vi "Node - Runtime Type Cast.vi"(8 "error in (no error)":errorcluster, 11 "Node Data In":T1) -> (0 "error out":errorcluster, 2 "Buffer Offset Out":u64, 3 "Node Data Out":T1)   [LabVIEW 2016, in "PXImc Router.lvlib"]
uses:
  Controls/Node Data.ctl
  <vilib>/NI Veristand/VeriStand Data/Byte Buffer/Byte Buffer.lvclass
  Controls/Node/Node - PXImc Parameters.ctl
  Controls/Node/Transfer Data.ctl
  Controls/Node/Node Ch Properties.ctl
  Controls/Data Type.ctl
  <vilib>/NI Veristand/VeriStand Data/Byte Buffer/Byte Buffer.lvclass/Byte Buffer.ctl
  <vilib>/NI Veristand/VeriStand Data/Type Conversion/Type Conversion.From Double (Boolean).vi
  <vilib>/NI Veristand/VeriStand Data/Byte Buffer/Byte Buffer.Write (Boolean).vi
  <vilib>/NI Veristand/VeriStand Data/Type Conversion/Type Conversion.From Double (SGL).vi
  <vilib>/NI Veristand/VeriStand Data/Byte Buffer/Byte Buffer.Write (SGL).vi
  <vilib>/NI Veristand/VeriStand Data/Byte Buffer/Byte Buffer.Write (DBL).vi
  <vilib>/NI Veristand/VeriStand Data/Type Conversion/Type Conversion.From Double (I8).vi
  <vilib>/NI Veristand/VeriStand Data/Byte Buffer/Byte Buffer.Write (I8).vi
  <vilib>/NI Veristand/VeriStand Data/Type Conversion/Type Conversion.From Double (I16).vi
  <vilib>/NI Veristand/VeriStand Data/Byte Buffer/Byte Buffer.Write (I16).vi
  <vilib>/NI Veristand/VeriStand Data/Type Conversion/Type Conversion.From Double (I32).vi
  <vilib>/NI Veristand/VeriStand Data/Byte Buffer/Byte Buffer.Write (I32).vi
  <vilib>/NI Veristand/VeriStand Data/Type Conversion/Type Conversion.From Double (I64).vi
  <vilib>/NI Veristand/VeriStand Data/Byte Buffer/Byte Buffer.Write (I64).vi
  <vilib>/NI Veristand/VeriStand Data/Type Conversion/Type Conversion.From Double (U8).vi
  <vilib>/NI Veristand/VeriStand Data/Byte Buffer/Byte Buffer.Write (U8).vi
  <vilib>/NI Veristand/VeriStand Data/Type Conversion/Type Conversion.From Double (U16).vi
  <vilib>/NI Veristand/VeriStand Data/Byte Buffer/Byte Buffer.Write (U16).vi
  <vilib>/NI Veristand/VeriStand Data/Type Conversion/Type Conversion.From Double (U32).vi
  <vilib>/NI Veristand/VeriStand Data/Byte Buffer/Byte Buffer.Write (U32).vi
  <vilib>/NI Veristand/VeriStand Data/Type Conversion/Type Conversion.From Double (U64).vi
  <vilib>/NI Veristand/VeriStand Data/Byte Buffer/Byte Buffer.Write (U64).vi
  <vilib>/NI Veristand/VeriStand Data/Byte Buffer/Byte Buffer.Write (String).vi
  <vilib>/NI Veristand/VeriStand Data/Byte Buffer/Byte Buffer.Subset.Set.vi
  <vilib>/NI Veristand/VeriStand Data/Byte Buffer/Byte Buffer.Get Buffer Pointer.vi
  <vilib>/NI Veristand/VeriStand Data/Byte Buffer/Byte Buffer.Get Buffer Size.vi
  <vilib>/NI Veristand/VeriStand Data/Memory Management/Memory Management.MoveByteBlock.Read (String).vi
  <vilib>/NI Veristand/VeriStand Data/Byte Buffer/Byte Buffer.Get Byte Order.vi
  <vilib>/NI Veristand/VeriStand Data/Memory Management/Memory Management.Handle Return.vi
  PXImc Router.lvlib
  <vilib>/NI Veristand/VeriStand Data/VeriStand Data.lvlib
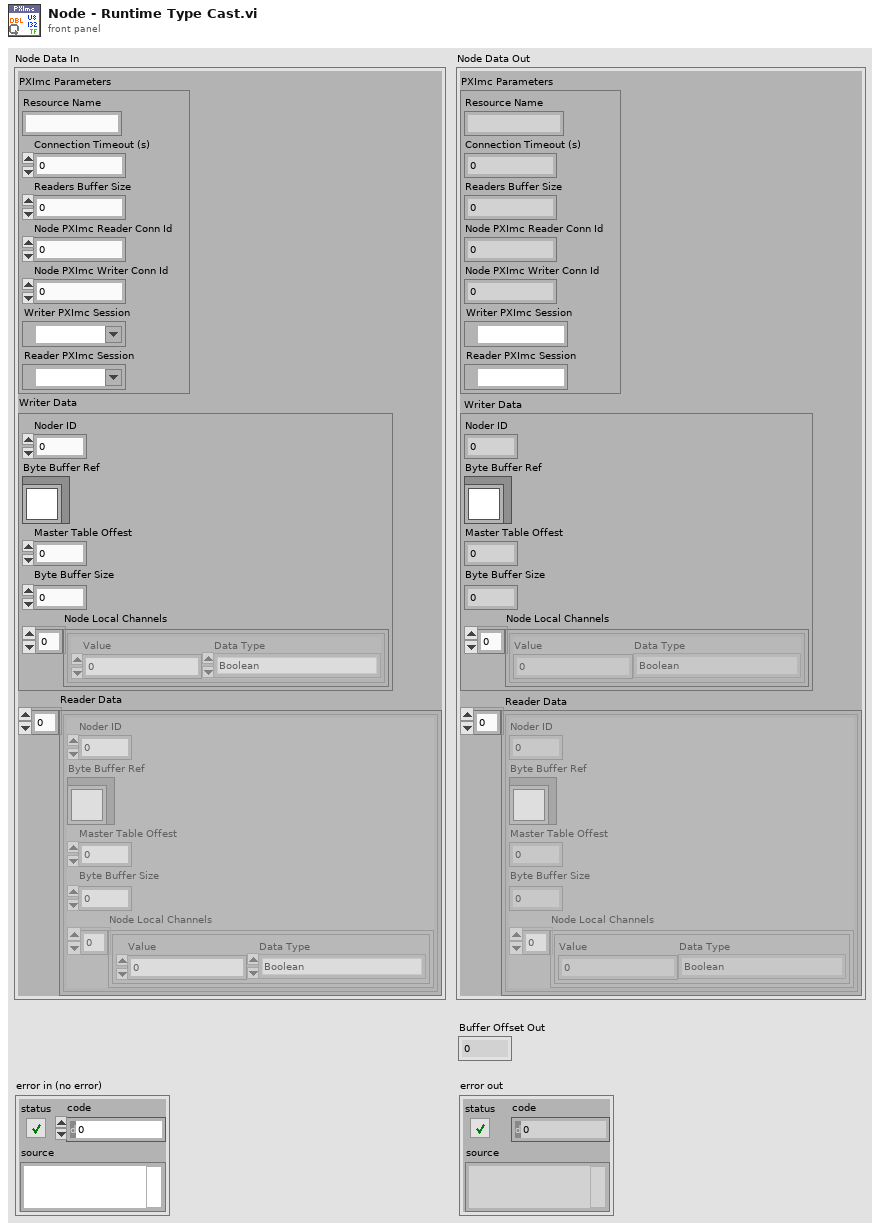
[diagram p1: front panel]
types:
  T1 = typedef "PXImc Router.lvlib/Node Data.ctl" = cluster{"PXImc Parameters":T2, "Writer Data":T3, "Reader Data":T3[]}
  T2 = typedef "PXImc Router.lvlib/Node - PXImc Parameters.ctl" = cluster{"Resource Name":string, "Connection Timeout (s)":dbl, "Readers Buffer Size":u32, "Node PXImc Reader Conn Id":u16, "Node PXImc Writer Conn Id":u16, "Writer PXImc Session":refnum<k21>, "Reader PXImc Session":refnum<k21>}
  T3 = typedef "PXImc Router.lvlib/Transfer Data.ctl" = cluster{"Noder ID":u32, "Byte Buffer Ref":refnum<class "Byte Buffer.lvclass">, "Master Table Offest":u32, "Byte Buffer Size":u32, "Node Local Channels":T4[]}
  T4 = typedef "PXImc Router.lvlib/Node Ch Properties.ctl" = cluster{"Value":dbl, "Data Type":T5}
  T5 = typedef "PXImc Router.lvlib/Data Type.ctl" = enum16{"Boolean", "SGL", "DBL", "I8", "I16", "I32", "I64", "U8", "U16", "U32", "U64"}
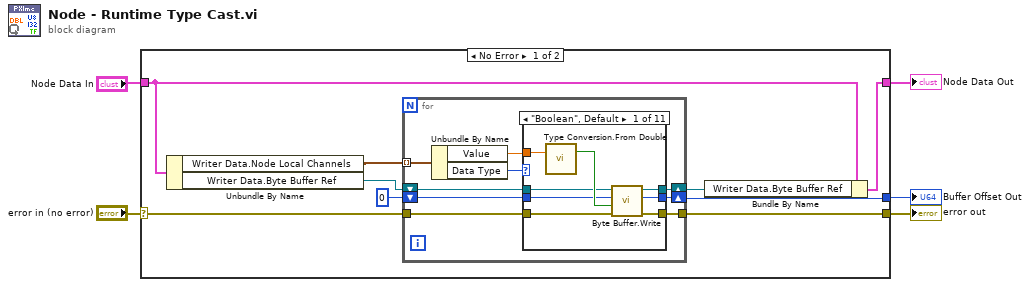
[diagram p0: block diagram]
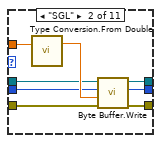
[diagram p2: hidden frame]
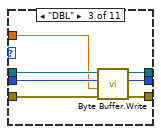
[diagram p3: hidden frame]
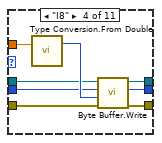
[diagram p4: hidden frame]
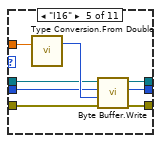
[diagram p5: hidden frame]
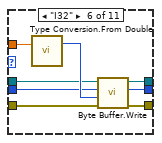
[diagram p6: hidden frame]
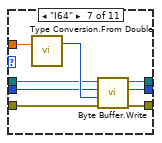
[diagram p7: hidden frame]
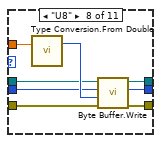
[diagram p8: hidden frame]
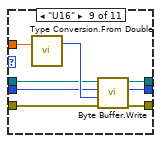
[diagram p9: hidden frame]
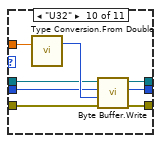
[diagram p10: hidden frame]
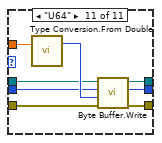
[diagram p11: hidden frame]
diagram:
  n1 = case shown="No Error" "error in (no error)" {
    selector: "error in (no error)" -> [w10 w111]
    tunnel: "Node Data In" -> [w14 w112]
    tunnel: [w13 w112] -> w4
    tunnel: [w11 w111] -> w2
    tunnel: [w6 _] -> w1
    frame No Error {
      n2 = Unbundle By Name(w14) -> ("Writer Data.Node Local Channels"=w7:T4[], "Writer Data.Byte Buffer Ref"=w9:refnum<class "Byte Buffer.lvclass">)
      n3 = for {
        tunnel: [w22] -> w11
        shift-right: [w23] -> w8
        shift-left: w9 -> [w21]
        shift-right: [w20] -> w6
        shift-left: u64 0 ("new buffer offset") -> [w19]
        tunnel: w10 -> [w18]
        tunnel: w7 -> [w17] mode=indexing
        n4 = Unbundle By Name(w17) -> ("Value"=w15:dbl, "Data Type"=w16:T5)
        n5 = case shown="\"Boolean\", Default" w16 {
          tunnel: [w30 w38 w46 w53 w61 w69 w77 w85 w93 w101 w109] -> w23
          tunnel: [w29 w37 w45 w52 w60 w68 w76 w84 w92 w100 w108] -> w22
          tunnel: w15 -> [w28 w36 w40 w51 w59 w67 w75 w83 w91 w99 w107]
          tunnel: w21 -> [w27 w35 w44 w50 w58 w66 w74 w82 w90 w98 w106]
          tunnel: [w26 w34 w43 w49 w57 w65 w73 w81 w89 w97 w105] -> w20
          tunnel: w19 -> [w24 w33 w42 w48 w56 w64 w72 w80 w88 w96 w104]
          tunnel: w18 -> [w25 w32 w41 w47 w55 w63 w71 w79 w87 w95 w103]
          frame "Boolean", Default {
            n6 = call-poly <vilib>:"Type Conversion.From Double.vi"("value in"=w28) -> ("value out"=w31:bool)  [unwired: 2 in]
            n7 = call-poly <vilib>:"Byte Buffer.Write.vi"("error in (no error)"=w25, "value"=w31, "buffer offset"=w24, "Byte Buffer in"=w27) -> ("error out"=w29:errorcluster, "new buffer offset"=w26:u64, "Byte Buffer out"=w30:refnum<class "Byte Buffer.lvclass">)  [unwired: 5 in]
          }
          frame "SGL" {
            n8 = call-poly <vilib>:"Type Conversion.From Double.vi"("value in"=w36) -> ("value out"=w39:sgl)  [unwired: 2 in]
            n9 = call-poly <vilib>:"Byte Buffer.Write.vi"("error in (no error)"=w32, "value"=w39, "buffer offset"=w33, "Byte Buffer in"=w35) -> ("error out"=w37:errorcluster, "new buffer offset"=w34:u64, "Byte Buffer out"=w38:refnum<class "Byte Buffer.lvclass">)  [unwired: 5 in]
          }
          frame "DBL" {
            n10 = call-poly <vilib>:"Byte Buffer.Write.vi"("error in (no error)"=w41, "value"=w40, "buffer offset"=w42, "Byte Buffer in"=w44) -> ("error out"=w45:errorcluster, "new buffer offset"=w43:u64, "Byte Buffer out"=w46:refnum<class "Byte Buffer.lvclass">)  [unwired: 5 in]
          }
          frame "I8" {
            n11 = call-poly <vilib>:"Type Conversion.From Double.vi"("value in"=w51) -> ("value out"=w54:i8)  [unwired: 2 in]
            n12 = call-poly <vilib>:"Byte Buffer.Write.vi"("error in (no error)"=w47, "value"=w54, "buffer offset"=w48, "Byte Buffer in"=w50) -> ("error out"=w52:errorcluster, "new buffer offset"=w49:u64, "Byte Buffer out"=w53:refnum<class "Byte Buffer.lvclass">)  [unwired: 5 in]
          }
          frame "I16" {
            n13 = call-poly <vilib>:"Type Conversion.From Double.vi"("value in"=w59) -> ("value out"=w62:i16)  [unwired: 2 in]
            n14 = call-poly <vilib>:"Byte Buffer.Write.vi"("error in (no error)"=w55, "value"=w62, "buffer offset"=w56, "Byte Buffer in"=w58) -> ("error out"=w60:errorcluster, "new buffer offset"=w57:u64, "Byte Buffer out"=w61:refnum<class "Byte Buffer.lvclass">)  [unwired: 5 in]
          }
          frame "I32" {
            n15 = call-poly <vilib>:"Type Conversion.From Double.vi"("value in"=w67) -> ("value out"=w70:i32)  [unwired: 2 in]
            n16 = call-poly <vilib>:"Byte Buffer.Write.vi"("error in (no error)"=w63, "value"=w70, "buffer offset"=w64, "Byte Buffer in"=w66) -> ("error out"=w68:errorcluster, "new buffer offset"=w65:u64, "Byte Buffer out"=w69:refnum<class "Byte Buffer.lvclass">)  [unwired: 5 in]
          }
          frame "I64" {
            n17 = call-poly <vilib>:"Type Conversion.From Double.vi"("value in"=w75) -> ("value out"=w78:i64)  [unwired: 2 in]
            n18 = call-poly <vilib>:"Byte Buffer.Write.vi"("error in (no error)"=w71, "value"=w78, "buffer offset"=w72, "Byte Buffer in"=w74) -> ("error out"=w76:errorcluster, "new buffer offset"=w73:u64, "Byte Buffer out"=w77:refnum<class "Byte Buffer.lvclass">)  [unwired: 5 in]
          }
          frame "U8" {
            n19 = call-poly <vilib>:"Type Conversion.From Double.vi"("value in"=w83) -> ("value out"=w86:u8)  [unwired: 2 in]
            n20 = call-poly <vilib>:"Byte Buffer.Write.vi"("error in (no error)"=w79, "value"=w86, "buffer offset"=w80, "Byte Buffer in"=w82) -> ("error out"=w84:errorcluster, "new buffer offset"=w81:u64, "Byte Buffer out"=w85:refnum<class "Byte Buffer.lvclass">)  [unwired: 5 in]
          }
          frame "U16" {
            n21 = call-poly <vilib>:"Type Conversion.From Double.vi"("value in"=w91) -> ("value out"=w94:u16)  [unwired: 2 in]
            n22 = call-poly <vilib>:"Byte Buffer.Write.vi"("error in (no error)"=w87, "value"=w94, "buffer offset"=w88, "Byte Buffer in"=w90) -> ("error out"=w92:errorcluster, "new buffer offset"=w89:u64, "Byte Buffer out"=w93:refnum<class "Byte Buffer.lvclass">)  [unwired: 5 in]
          }
          frame "U32" {
            n23 = call-poly <vilib>:"Type Conversion.From Double.vi"("value in"=w99) -> ("value out"=w102:u32)  [unwired: 2 in]
            n24 = call-poly <vilib>:"Byte Buffer.Write.vi"("error in (no error)"=w95, "value"=w102, "buffer offset"=w96, "Byte Buffer in"=w98) -> ("error out"=w100:errorcluster, "new buffer offset"=w97:u64, "Byte Buffer out"=w101:refnum<class "Byte Buffer.lvclass">)  [unwired: 5 in]
          }
          frame "U64" {
            n25 = call-poly <vilib>:"Type Conversion.From Double.vi"("value in"=w107) -> ("value out"=w110:u64)  [unwired: 2 in]
            n26 = call-poly <vilib>:"Byte Buffer.Write.vi"("error in (no error)"=w103, "value"=w110, "buffer offset"=w104, "Byte Buffer in"=w106) -> ("error out"=w108:errorcluster, "new buffer offset"=w105:u64, "Byte Buffer out"=w109:refnum<class "Byte Buffer.lvclass">)  [unwired: 5 in]
          }
        }
      }
      n27 = Bundle By Name(cluster=w14, "Writer Data.Byte Buffer Ref"=w8) -> (w13:T1)
    }
    frame Error {
    }
  }
  "error out" <- w2
  "Node Data Out" <- w4
  "Buffer Offset Out" <- w1
